vi "Param_Analysis.vi"(7 "error in (no error)":errorcluster, 8 "Data Folder":path=path "D:/Userdata/Documents/Lab/8_26/diF-TES ADT 0_33pct cB_SAC-Shaker/data", 9 "Parameter String":string, 10 "Parameter Name":string, 11 "Stats Folder":path=path "D:/Userdata/Documents/Lab/8_26/diF-TES ADT 0_33pct cB_SAC-Shaker/data") -> (0 "Output File":path=path "D:/Userdata/Documents/Lab/8_26/diF-TES ADT 0_33pct cB_SAC-Shaker/data", 1 "error out":errorcluster, 2 "Histogram Array":string[](array[string]), 3 "Param vs L Array":string[][](array[string]))   [LabVIEW 2011]
doc: "Stats Folder - Directory where the analysis is to be stored\n\nData Folder - Directory where the files to be analyzed are stored\n\nParameter Name - String to be used as the name of the outputed file for the analyzed paramters \n\nParameter String - String that should be identically equal to the name adjacent to the parameter to be analyzed in the data files\n\n\nOutput File - Directory where the analysis summary is located"
uses:
  <vilib>/Utility/file.llb/Write To Spreadsheet File (string).vi
  <vilib>/Utility/file.llb/Read From Spreadsheet File (string).vi
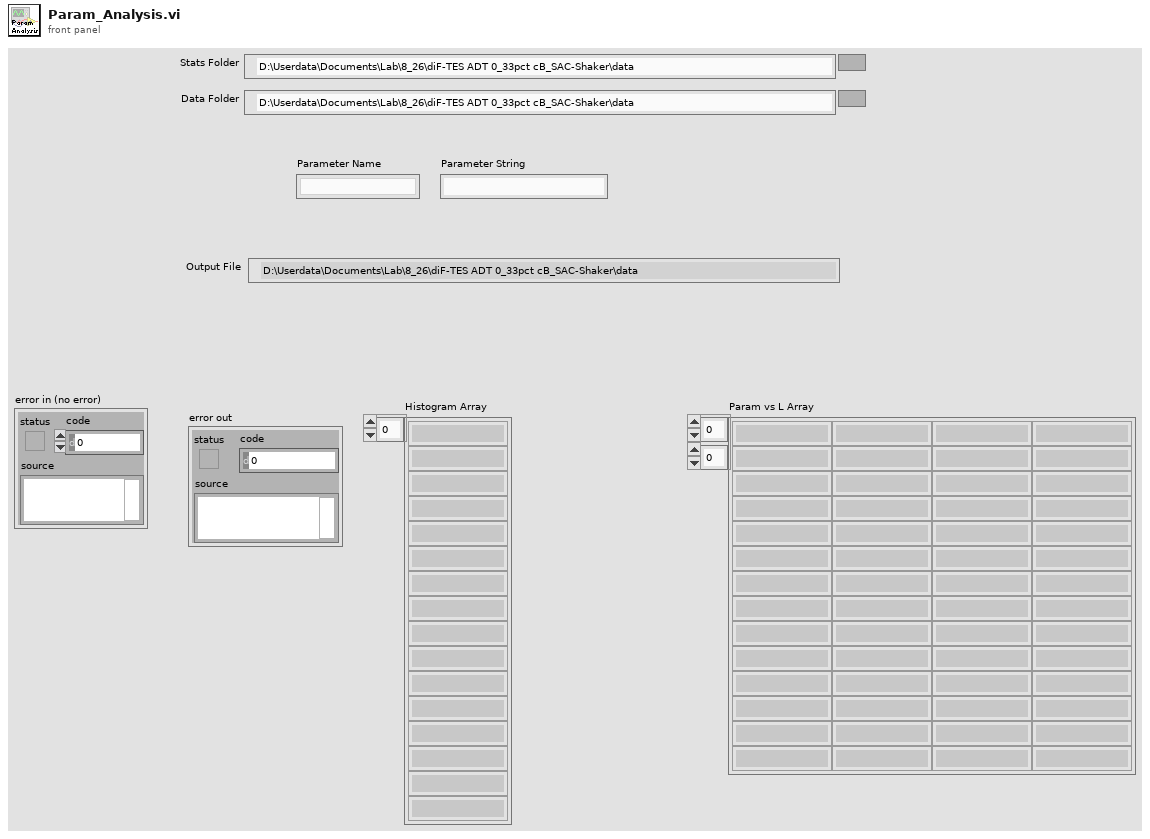
[diagram p1: front panel]
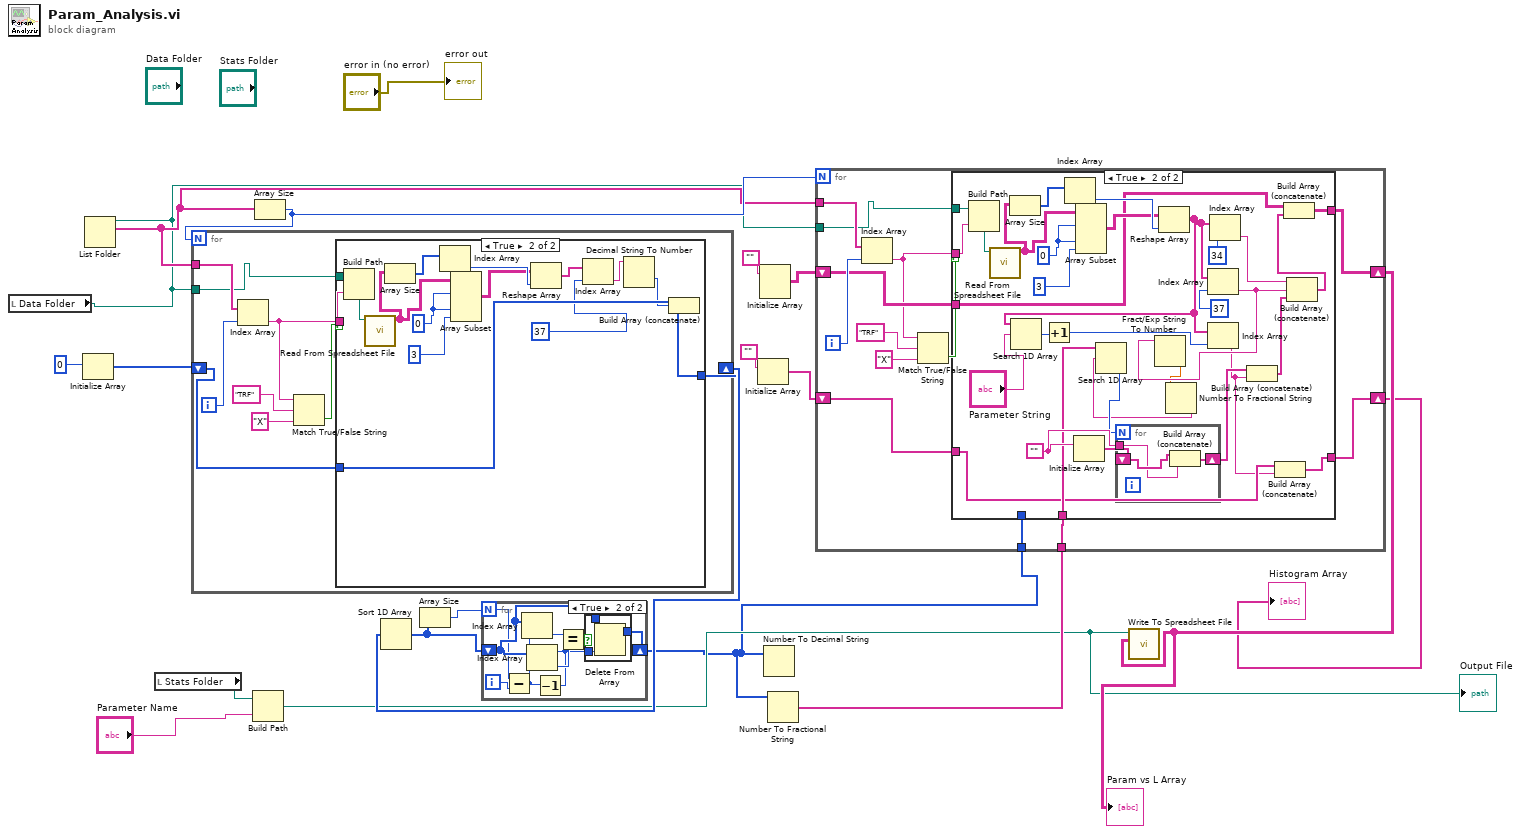
[diagram p0: block diagram]
diagram:
  n1 = local read "Data Folder"() -> (w1:path)
  n2 = Initialize Array(0) -> (w12:i32[])  [unwired: 1 in]
  n3 = List Folder(path=w1) -> (filenames=w19:string[])  [unwired: 3 in, 3 out]
  n4 = local read "Stats Folder"() -> (w9:path)
  n5 = Build Path(base path=w9, name or relative path="Parameter Name") -> (appended path=w8:path)
  "Output File" <- w8
  n6 = Array Size(array=w19) -> (size(s)=w20:i32)
  n7 = for {
    N: w20 -> [_]
    tunnel: w19 -> [w29]
    tunnel: w1 -> [w27]
    shift-right: [w22] -> w18
    shift-left: w12 -> [w21]
    i -> [w28]
    n8 = Index Array(array=w29, index=w28) -> (element=w26:string)
    n9 = Match True/False String(2:"X", 3:"TRF", 4:w26) -> (0:w24:bool)  [unwired: 1 out]
    n10 = case shown="True" w24 {
      tunnel: w27 -> [_ w45]
      tunnel: w26 -> [_ w37]
      tunnel: [w30 w36] -> w22
      tunnel: w21 -> [w30 w35]
      frame False {
      }
      frame True {
        w42 = 0
        n11 = Build Path(base path=w45, name or relative path=w37) -> (appended path=w44:path)
        n12 = call-poly <vilib>:"Read From Spreadsheet File.vi"("file path (dialog if empty)"=w44) -> ("all rows"=w40:string[][])  [unwired: 6 in, 4 out]
        n13 = Array Size(array=w40) -> (size(s)=w41:i32[])
        n14 = Index Array(array=w41) -> (element=w39:i32)  [unwired: 1 in]
        n15 = Array Subset(array=w40, index (row)=w42, index (col)=w42, length (col)=3) -> (w38:string[][])  [unwired: 1 in]
        n16 = Reshape Array(w38, w39) -> (w32:string[])
        n17 = Index Array(array=w32, index=37) -> (element=w34:string)
        n18 = Decimal String To Number(string=w34) -> (number=w33:i32)  [unwired: 2 in, 1 out]
        n19 = Build Array (concatenate)(w35, w33) -> (w36:i32[])
      }
    }
  }
  n20 = Sort 1D Array(array=w18) -> (sorted array=w17:i32[])
  n21 = Array Size(array=w17) -> (size(s)=w16:i32)
  n22 = for {
    N: w16 -> [w49]
    shift-right: [w46] -> w6
    shift-left: w17 -> [w51]
    i -> [w50]
    n23 = Subtract(x=w49, y=w50) -> (x-y=w48:i32)
    n24 = Index Array(array=w51, index=w48) -> (element=w53:i32)
    n25 = Decrement(x=w48) -> (x-1=w47:i32)
    n26 = Index Array(array=w51, index=w47) -> (element=w54:i32)
    n27 = Equal?(x=w53, y=w54) -> (x = y?=w52:bool)
    n28 = case shown="True" w52 {
      tunnel: w51 -> [w55 w58]
      tunnel: w47 -> [_ w57]
      tunnel: [w55 w56] -> w46
      frame False {
      }
      frame True {
        n29 = Delete From Array(array=w58, index=w57) -> (array with subset deleted=w56:i32[])  [unwired: 1 in, 1 out]
      }
    }
  }
  n30 = Initialize Array("") -> (w3:string[])  [unwired: 1 in]
  n31 = Initialize Array("") -> (w5:string[][])  [unwired: 2 in]
  n32 = Number To Decimal String(number=w6) -> ()  [unwired: 1 in, 1 out]
  n33 = Number To Fractional String(number=w6) -> (F-format string=w10:string[])  [unwired: 3 in]
  n34 = for {
    N: w20 -> [_]
    tunnel: w19 -> [w71]
    tunnel: w1 -> [w69]
    shift-right: [w67] -> w11
    shift-left: w5 -> [w68]
    tunnel: w10 -> [w62]
    tunnel: w6 -> [w61]
    shift-right: [w59] -> w2
    shift-left: w3 -> [w60]
    i -> [w70]
    n35 = Index Array(array=w71, index=w70) -> (element=w66:string)
    n36 = Match True/False String(2:"X", 3:"TRF", 4:w66) -> (0:w64:bool)  [unwired: 1 out]
    n37 = case shown="True" w64 {
      tunnel: w69 -> [_ w104]
      tunnel: w68 -> [w73 w94]
      tunnel: [w73 w92] -> w67
      tunnel: w66 -> [_ w91]
      tunnel: w62 -> [_ w77]
      tunnel: w61 -> [_ _]
      tunnel: w60 -> [w72 w75]
      tunnel: [w72 w76] -> w59
      frame False {
      }
      frame True {
        w86 = ""
        w101 = 0
        n38 = Build Path(base path=w104, name or relative path=w91) -> (appended path=w103:path)
        n39 = call-poly <vilib>:"Read From Spreadsheet File.vi"("file path (dialog if empty)"=w103) -> ("all rows"=w99:string[][])  [unwired: 6 in, 4 out]
        n40 = Array Size(array=w99) -> (size(s)=w100:i32[])
        n41 = Index Array(array=w100) -> (element=w98:i32)  [unwired: 1 in]
        n42 = Initialize Array(w86) -> (w87:string[])  [unwired: 1 in]
        n43 = Array Subset(array=w99, index (row)=w101, index (col)=w101, length (col)=3) -> (w97:string[][])  [unwired: 1 in]
        n44 = Reshape Array(w97, w98) -> (w83:string[])
        n45 = Search 1D Array(1D array=w83, element="Parameter String") -> (index of element=w84:i32)  [unwired: 1 in]
        n46 = Increment(x=w84) -> (x+1=w82:i32)
        n47 = Index Array(array=w83, index=37) -> (element=w80:string)
        n48 = Fract/Exp String To Number(string=w80) -> (number=w79:dbl)  [unwired: 3 in, 1 out]
        n49 = Number To Fractional String(number=w79) -> (F-format string=w78:string)  [unwired: 3 in]
        n50 = Search 1D Array(1D array=w77, element=w78) -> (index of element=w85:i32)  [unwired: 1 in]
        n51 = for {
          N: w85 -> [_]
          shift-right: [w106] -> w89
          shift-left: w87 -> [w107]
          tunnel: w86 -> [w105]
          n52 = Build Array (concatenate)(w107, w105) -> (w106:string[])
        }
        n53 = Index Array(array=w83, index=w82) -> (element=w74:string)
        n54 = Index Array(array=w83, index=34) -> (element=w90:string)
        n55 = Build Array (concatenate)(w89, w74) -> (w88:string[])
        n56 = Build Array (concatenate)(w75, w74) -> (w76:string[])
        n57 = Build Array (concatenate)(w90, w80, w88) -> (w93:string[])
        n58 = Build Array (concatenate)(w94, w93) -> (w92:string[][])
      }
    }
  }
  "Param vs L Array" <- w11
  "Histogram Array" <- w2
  n59 = call-poly <vilib>:"Write To Spreadsheet File.vi"("2D data"=w11, "file path (dialog if empty)"=w8) -> ()  [unwired: 6 in, 1 out]
  "error out" <- "error in (no error)"
